vi "AI-Motor_Set.vi"(8 "Error In":errorcluster, 11 "Motor ID (0)":u8) -> (0 "Error Out":errorcluster)   [LabVIEW 2019]
uses:
  <instrlib>/Dynamixel Motor/Public/Motor Operation/Low Level/Baud Setting.ctl
  Variable/Position.vi
  <instrlib>/Dynamixel Motor/Dynamixel Motor.lvlib
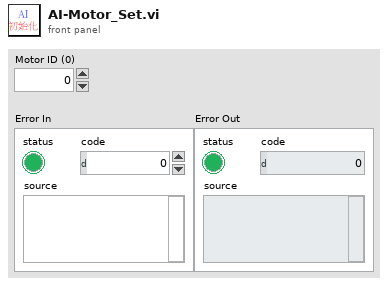
[diagram p1: front panel]
types:
  T1 = typedef "Dynamixel Motor.lvlib/Baud Setting.ctl" = u8
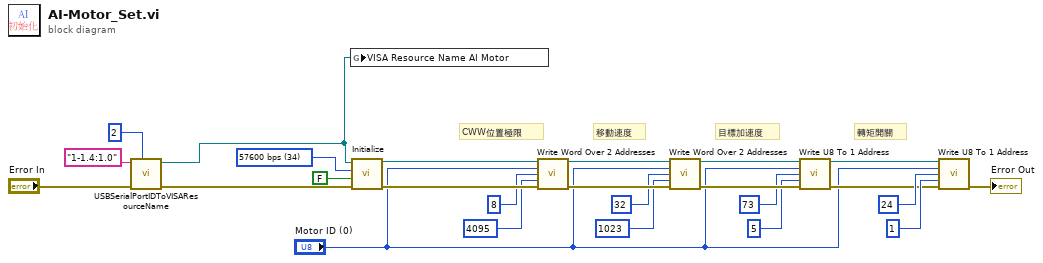
[diagram p0: block diagram]
diagram:
  w23 = T1 34 items=["1,000,000 bps"=1, "500,000 bps"=3, "400,000 bps"=4, "250,000 bps"=7, "200,000 bps"=9, "115200 bps"=16, "57600 bps"=34, "19200 bps"=103, "9600 bps"=207] ("Baud rate (57600 bps)")
  # "轉矩開關"
  # "目標加速度"
  # "移動速度"
  # "CWW位置極限"
  n1 = call "USBSerialPortIDToVISAResourceName.vi"("搜索有效數量"=u32 2, "Error In"="Error In", "端口號"="1-1.4:1.0") -> ("Error Out"=w4:errorcluster, "VISA Resource Name"=w2:refnum<visa-resource-name>)  [unwired: 7 in]
  n2 = global write "Position.vi" "VISA Resource Name AI Motor"(w2) -> ()
  n3 = call <instrlib>:"Initialize.vi"("error in (no error)"=w4, "Force Baud Rate (True)"=FALSE, "Baud rate (57600 bps)"=w23, "VISA resource name"=w2) -> ("error out"=w24:errorcluster, "VISA resource name out"=w20:refnum<visa-resource-name>)  [unwired: 6 in]
  n4 = call <instrlib>:"Write Word Over 2 Addresses.vi"("VISA resource name"=w20, "Motor ID (0)"="Motor ID (0)", "Address number (0)"=u8 8, "Parameter (0)"=u16 4095, "error in (no error)"=w24) -> ("VISA resource name out"=w17:refnum<visa-resource-name>, "error out"=w25:errorcluster)  [unwired: 9 in]
  n5 = call <instrlib>:"Write Word Over 2 Addresses.vi"("VISA resource name"=w17, "Motor ID (0)"="Motor ID (0)", "Address number (0)"=u8 32, "Parameter (0)"=u16 1023, "error in (no error)"=w25) -> ("VISA resource name out"=w12:refnum<visa-resource-name>, "error out"=w15:errorcluster)  [unwired: 9 in]
  n6 = call <instrlib>:"Write U8 To 1 Address.vi"("VISA resource name"=w12, "Motor ID (0)"="Motor ID (0)", "Address number (0)"=u8 73, "Parameter (0)"=u16 5, "error in (no error)"=w15) -> ("VISA resource name out"=w8:refnum<visa-resource-name>, "error out"=w9:errorcluster)  [unwired: 9 in]
  n7 = call <instrlib>:"Write U8 To 1 Address.vi"("VISA resource name"=w8, "Motor ID (0)"="Motor ID (0)", "Address number (0)"=u8 24, "Parameter (0)"=u16 1, "error in (no error)"=w9) -> ("error out"=→"Error Out":errorcluster)  [unwired: 9 in, 1 out]
